vi "OAT Resampled Signal Slow Roll Baseline.vi"(4 "average revolution":i32, 6 "slow roll\nrevolution number":i32, 7 "reset? (True)":bool=TRUE, 8 "error in (no error)":errorcluster, 10 "baseline in":cluster{"r0":dbl, "dr":dbl, "Y":dbl[]}={"r0"=0.0, "dr"=1.0, "Y"=[]} {"r0" format="%.2p"; "dr" format="%.2p"; "Y" format="%.2f"}, 11 "resampled signal in":cluster{"r0":dbl, "dr":dbl, "Y":dbl[]}={"r0"=0.0, "dr"=1.0, "Y"=[]} {"r0" format="%.2p"; "dr" format="%.2p"; "Y" format="%.2f"}) -> (0 "error out":errorcluster, 2 "baseline out":cluster{"r0":dbl, "dr":dbl, "Y":dbl[]}={"r0"=0.0, "dr"=1.0, "Y"=[]} {"r0" format="%.2p"; "dr" format="%.2p"; "Y" format="%.2f"}, 3 "resampled signal out":cluster{"r0":dbl, "dr":dbl, "Y":dbl[]}={"r0"=0.0, "dr"=1.0, "Y"=[]} {"r0" format="%.2p"; "dr" format="%.2p"; "Y" format="%.2f"})   [LabVIEW 2017, in "SoundVib_Resampling.lvlib"]
uses:
  <vilib>/addons/Sound and Vibration/Order Analysis/Resample Order Tracking/SoundVib_Resampling.lvlib
  <vilib>/addons/Sound and Vibration/Order Analysis/Resample Order Tracking/SubVIs/OAT Verify Resampled Signal (Single Channel).vi
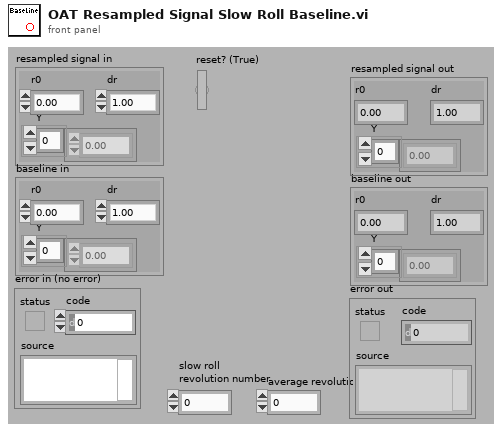
[diagram p1: front panel]
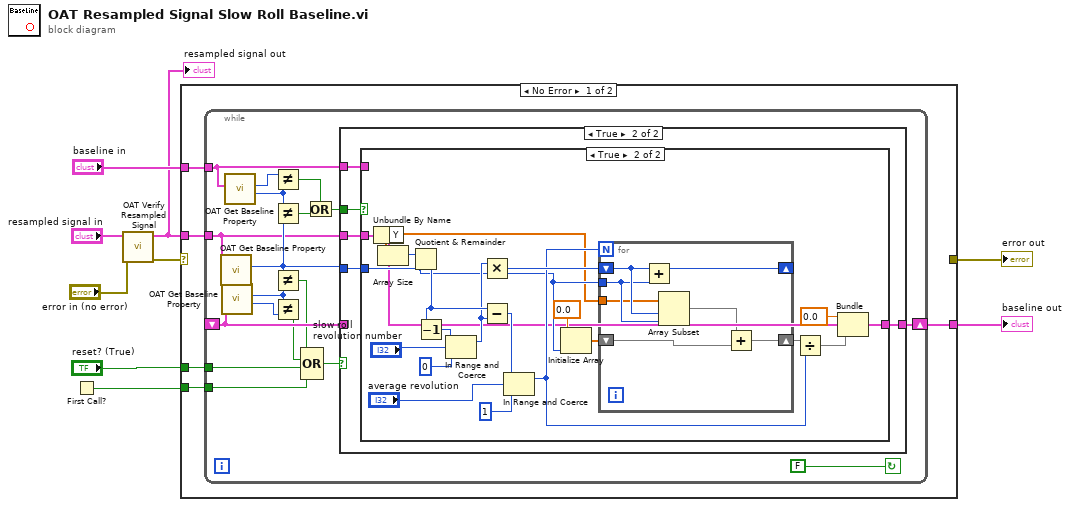
[diagram p0: block diagram]
diagram:
  n1 = First Call?() -> (First Call?: T/F=w4:bool)
  n2 = call-poly <vilib>:"OAT Verify Resampled Signal.vi"("error in (no error)"="error in (no error)", "resampled signal"="resampled signal in") -> ("error out"=w6:errorcluster, "resampled signal dup"=w1:cluster{"r0":dbl, "dr":dbl, "Y":dbl[]})  [unwired: 7 in, 1 out]
  "resampled signal out" <- w1
  n3 = case shown="No Error" w6 {
    selector: w6 -> [_ w68]
    tunnel: [w13 w67] -> w9
    tunnel: w1 -> [w14 _]
    tunnel: [_ w68] -> w5
    tunnel: w4 -> [w12 _]
    tunnel: "reset? (True)" -> [w11 _]
    tunnel: "baseline in" -> [w10 w67]
    frame No Error {
      n4 = while {
        tunnel: w14 -> [w15]
        shift-right: [w32] -> w13
        shift-left: _ -> [w26]
        tunnel: w12 -> [w29]
        tunnel: w11 -> [w28]
        tunnel: w10 -> [w22]
        stop <- FALSE continue-if-true
        n5 = call <vilib>:"OAT Get Baseline Property.vi"("baseline"=w15) -> ("samples/rev"=w19:i32)  [unwired: 9 in, 1 out]
        n6 = call <vilib>:"OAT Get Baseline Property.vi"("baseline"=w26) -> ("samples"=w30:i32, "samples/rev"=w24:i32)  [unwired: 9 in]
        n7 = call <vilib>:"OAT Get Baseline Property.vi"("baseline"=w22) -> ("samples"=w20:i32, "samples/rev"=w21:i32)  [unwired: 9 in]
        n8 = Not Equal?(x=w21, y=w20) -> (x != y?=w18:bool)
        n9 = Not Equal?(x=w20, y=w19) -> (x != y?=w17:bool)
        n10 = Not Equal?(x=w19, y=w24) -> (x != y?=w23:bool)
        n11 = Not Equal?(x=w24, y=w30) -> (x != y?=w25:bool)
        n12 = Compound Arithmetic op=OR(w23, w25, w28, w29) -> (w27:bool)
        n13 = Or(x=w18, y=w17) -> (x .or. y?=w16:bool)
        n14 = case shown="True" w27 {
          tunnel: [w33 w38] -> w32
          tunnel: w19 -> [_ w37]
          tunnel: w26 -> [w33 _]
          tunnel: w16 -> [_ w36]
          tunnel: w22 -> [_ w35]
          tunnel: w15 -> [_ w34]
          frame False {
          }
          frame True {
            n15 = case shown="True" w36 {
              tunnel: [w39 w42] -> w38
              tunnel: w37 -> [_ w47]
              tunnel: w35 -> [w39 _]
              tunnel: w34 -> [_ w44]
              frame False {
              }
              frame True {
                n16 = Unbundle By Name(w44) -> ("Y"=w40:dbl[])
                n17 = Array Size(array=w40) -> (size(s)=w54:i32)
                n18 = Quotient & Remainder(x=w54, y=w47) -> (floor(x/y)=w57:i32)  [unwired: 1 out]
                n19 = Decrement(x=w57) -> (x-1=w55:i32)
                n20 = In Range and Coerce(upper limit=w55, x="slow roll\nrevolution number", lower limit=0) -> (coerced(x)=w53:i32)  [unwired: 1 out]
                n21 = Multiply(x=w53, y=w47) -> (x*y=w52:i32)
                n22 = Subtract(x=w57, y=w53) -> (x-y=w58:i32)
                n23 = In Range and Coerce(upper limit=w58, x="average revolution", lower limit=1 ("y")) -> (coerced(x)=w48:i32)  [unwired: 1 out]
                n24 = Initialize Array(0.0 ("element"), w47) -> (w50:dbl[])
                n25 = for {
                  N: w48 -> [_]
                  shift-right: [w61] -> _
                  shift-left: w52 -> [w66]
                  tunnel: w47 -> [w65]
                  shift-right: [w63] -> w49
                  shift-left: w50 -> [w64]
                  tunnel: w40 -> [w62]
                  n26 = Add(x=w66, y=w65) -> (x+y=w61:i32)
                  n27 = Array Subset(array=w62, index=w66, length=w65) -> (w60:dbl[])
                  n28 = Add(x=w60, y=w64) -> (x+y=w63:dbl[])
                }
                n29 = Divide(x=w49, y=w48) -> (x/y=w43:dbl[])
                n30 = Bundle(cluster=w44, "r0"=0.0, "Y"=w43) -> (w42:cluster{"r0":dbl, "dr":dbl, "Y":dbl[]})  [unwired: 1 in]
              }
            }
          }
        }
      }
    }
    frame Error {
    }
  }
  "baseline out" <- w9
  "error out" <- w5
